vi "code+tester.vi"() -> ()   [LabVIEW 2020]
panel:
  in  "y offset":i32
  in  "x offiset":i32
  in  "core size":i32
  in  "dim 2":i32
  in  "dim1":i32
  in  "error in (no error)":errorcluster
  out "error out":errorcluster
  out "return value":i32[](array[numeric])
  in  "module path":path
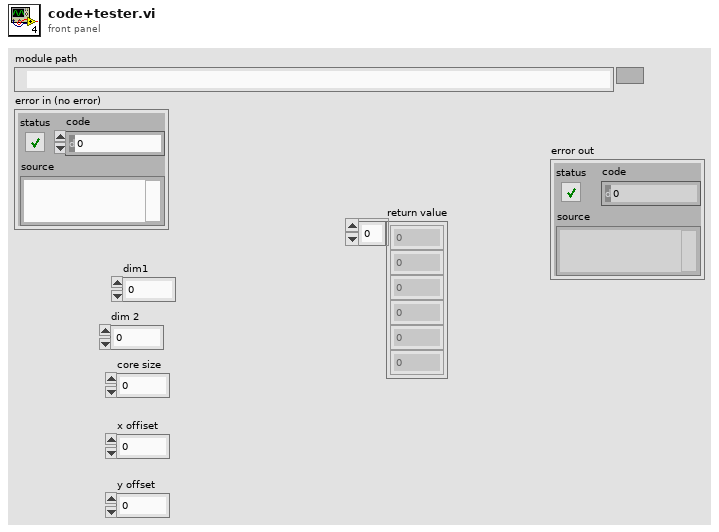
[diagram p1: front panel]
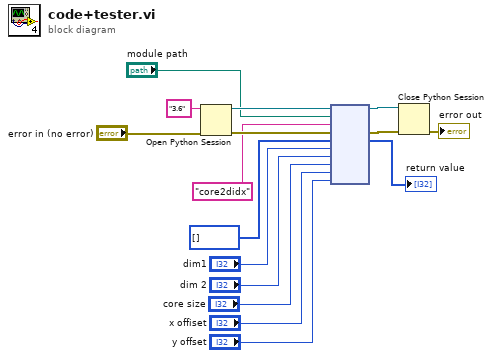
[diagram p0: block diagram]
diagram:
  n1 = Open Python Session(python version="3.6" ("Python version"), 3:"error in (no error)") -> (session out=w16:refnum<k35>, error out=w15:errorcluster)  [unwired: 1 in]
  n2 = node(w16, "module path", "core2didx" ("function name"), w15, i32[] [], "dim1", "dim 2", "core size", "x offiset", "y offset") -> (w14:refnum<k35>, w13:errorcluster, →"return value":i32[])  [unwired: 5 in, 2 out]
  n3 = Close Python Session(session in=w14, error in=w13) -> (11:→"error out":errorcluster)
